vi "Building Array.vi"(0 "Vy array":dbl[](array[numeric]), 1 "Vx array":dbl[](array[numeric]), 2 "Timepoints":dbl[](array[numeric]), 3 "Folder to Save":path, 4 "No. of Gr":i32, 5 "No. of Sets":i32, 6 "Name of File":string, 7 "Folder Name":string) -> ()   [LabVIEW 2014]
uses:
  <vilib>/Utility/file.llb/Write Delimited Spreadsheet (DBL).vi
  <vilib>/Utility/file.llb/Read Delimited Spreadsheet (DBL).vi
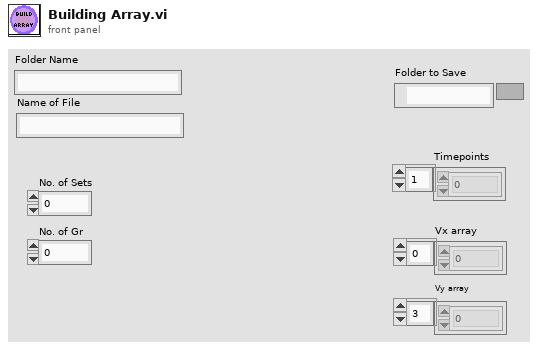
[diagram p1: front panel]
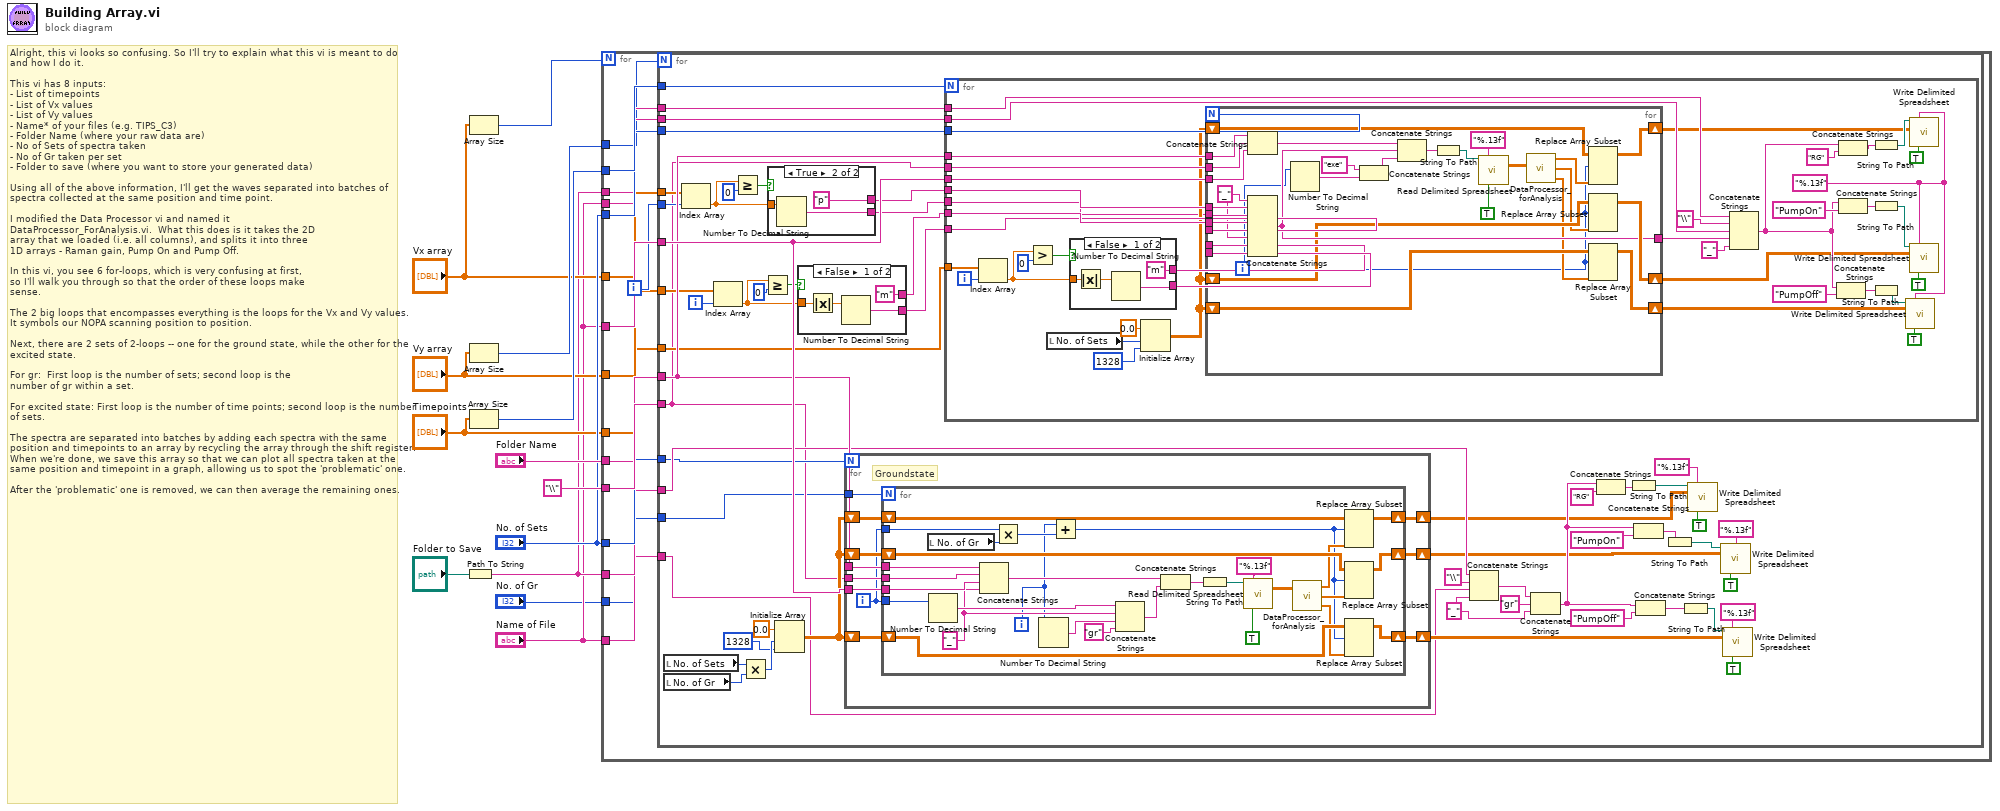
[diagram p0: block diagram]
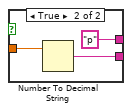
[diagram p2: hidden frame]
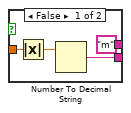
[diagram p3: hidden frame]
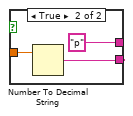
[diagram p4: hidden frame]
diagram:
  # "Alright, this vi looks so confusing. So I'll try to explain what this vi is meant to do and how I do it.\n\nThis vi has 8 inputs:\n- List of timepoints \n- List of Vx values \n- List of Vy values\n- Name* of your files (e.g. TIPS_C3)\n- Folder Name (where your raw data are)\n- No of Sets of spectra taken\n- No of Gr taken per set\n- Folder to save (where you want to store your generated data)\n\nUsing all of the above information, I'll get the waves separated into batches of spectra collected at the same position and time point.\n\nI modified the Data Processor vi and named it\nDataProcessor_ForAnalysis.vi.  What this does is it takes the 2D\narray that we loaded (i.e. all columns), and splits it into three\n1D arrays - Raman gain, Pump On and Pump Off.\n\nIn this vi, you see 6 for-loops, which is very confusing at first,\nso I'll walk you through so that the order of these loops make \nsense. \n\nThe 2 big loops that encompasses everything is the loops for the Vx and Vy values.  It symbols our NOPA scanning position to position.\n\nNext, there are 2 sets of 2-loops -- one for the ground state, while the other for the excited state.\n\nFor gr:  First loop is the number of sets; second loop is the\nnumber of gr within a set.\n\nFor excited state: First loop is the number of time points; second loop is the number of sets.\n\nThe spectra are separated into batches by adding each spectra with the same position and timepoints to an array by recycling the array through the shift register. When we're done, we save this array so that we can plot all spectra taken at the same position and timepoint in a graph, allowing us to spot the 'problematic' one. \n\nAfter the 'problematic' one is removed, we can then average the remaining ones."
  n1 = Path To String(path="Folder to Save") -> (string=w4:string)
  n2 = Array Size(array="Vx array") -> (size(s)=w2:i32)
  n3 = Array Size(array="Vy array") -> (size(s)=w11:i32)
  n4 = Array Size(array="Timepoints") -> (size(s)=w10:i32)
  n5 = for {
    N: w2 -> [_]
    tunnel: "Name of File" -> [w29]
    tunnel: "\\" -> [w28]
    tunnel: "Folder Name" -> [w27]
    tunnel: w11 -> [w15]
    tunnel: w10 -> [w26]
    tunnel: "No. of Sets" -> [w25]
    tunnel: "No. of Sets" -> [w24]
    tunnel: "Vx array" -> [w23]
    tunnel: "Vy array" -> [w21]
    tunnel: "Timepoints" -> [w20]
    tunnel: w4 -> [w19]
    tunnel: w4 -> [w18]
    tunnel: "Name of File" -> [w17]
    tunnel: "Name of File" -> [w16]
    tunnel: "No. of Gr" -> [w14]
    i -> [w22]
    n6 = for {
      N: w15 -> [_]
      tunnel: w29 -> [w84]
      tunnel: w28 -> [w36]
      tunnel: w27 -> [w83]
      tunnel: w26 -> [w82]
      tunnel: w25 -> [w81]
      tunnel: w24 -> [w39]
      tunnel: w23 -> [w77]
      tunnel: w22 -> [w78]
      tunnel: w21 -> [w73]
      tunnel: w20 -> [w67]
      tunnel: w19 -> [w66]
      tunnel: w18 -> [w65]
      tunnel: w17 -> [w32]
      tunnel: w16 -> [w49]
      tunnel: w14 -> [w35]
      i -> [w72]
      w45 = "_" ("string")
      n7 = local read "No. of Sets"() -> (w34:i32)
      n8 = local read "No. of Gr"() -> (w33:i32)
      n9 = Index Array(array=w77, index=w78) -> (element=w37:dbl)
      n10 = Index Array(array=w73, index=w72) -> (element=w74:dbl)
      n11 = Greater Or Equal?(x=w37, y=0) -> (x >= y?=w79:bool)
      n12 = Multiply(x=w34, y=w33) -> (x*y=w31:i32)
      n13 = Greater Or Equal?(x=w74, y=0) -> (x >= y?=w76:bool)
      n14 = case shown="True" w79 {
        tunnel: ["m" "p"] -> w71
        tunnel: w37 -> [w95 w96]
        tunnel: [w93 w97] -> w70
        frame False {
          n15 = Absolute Value(x=w95) -> (abs(x)=w94:dbl)
          n16 = Number To Decimal String(number=w94) -> (decimal integer string=w93:string)  [unwired: 1 in]
        }
        frame True {
          n17 = Number To Decimal String(number=w96) -> (decimal integer string=w97:string)  [unwired: 1 in]
        }
      }
      n18 = Initialize Array(0.0 ("element"), w31, 1328 ("dimension size")) -> (w38:dbl[][])
      n19 = case shown="False" w76 {
        tunnel: ["m" "p"] -> w69
        tunnel: w74 -> [w87 w89]
        tunnel: [w85 w90] -> w68
        frame False {
          n20 = Absolute Value(x=w87) -> (abs(x)=w86:dbl)
          n21 = Number To Decimal String(number=w86) -> (decimal integer string=w85:string)  [unwired: 1 in]
        }
        frame True {
          n22 = Number To Decimal String(number=w89) -> (decimal integer string=w90:string)  [unwired: 1 in]
        }
      }
      n23 = for {
        N: w39 -> [_]
        tunnel: w84 -> [w109]
        tunnel: w36 -> [w108]
        tunnel: w83 -> [w107]
        tunnel: w35 -> [w106]
        shift-right: [w105] -> w41
        shift-left: w38 -> [w102]
        shift-right: [w104] -> w43
        shift-left: w38 -> [w101]
        shift-right: [w103] -> w42
        shift-left: w38 -> [w100]
        i -> [w99]
        # "Groundstate"
        n24 = for {
          N: w106 -> [_]
          tunnel: w109 -> [w135]
          tunnel: w108 -> [w136]
          tunnel: w107 -> [w137]
          tunnel: w99 -> [w138]
          shift-right: [w119] -> w105
          shift-left: w102 -> [w118]
          shift-right: [w120] -> w103
          shift-left: w100 -> [w121]
          shift-right: [w123] -> w104
          shift-left: w101 -> [w122]
          tunnel: w99 -> [w116]
          i -> [w110]
          w133 = "_"
          n25 = local read "No. of Gr"() -> (w117:i32)
          n26 = Number To Decimal String(number=w138) -> (decimal integer string=w134:string)  [unwired: 1 in]
          n27 = Concatenate Strings(w137, w136, w135, w133) -> (w131:string)
          n28 = Multiply(x=w116, y=w117) -> (x*y=w115:i32)
          n29 = Number To Decimal String(number=w110) -> (decimal integer string=w132:string)  [unwired: 1 in]
          n30 = Add(x=w110, y=w115) -> (x+y=w111:i32)
          n31 = Concatenate Strings(w134, w133, w132, "gr" ("string")) -> (w124:string)
          n32 = Concatenate Strings(w131, w124) -> (w130:string)
          n33 = String To Path(string=w130) -> (path=w127:path)
          n34 = call-poly <vilib>:"Read Delimited Spreadsheet.vi"("file path (dialog if empty)"=w127, "format (%.3f)"="%.13f", "transpose? (F)"=TRUE) -> ("all rows"=w129:dbl[][])  [unwired: 7 in, 5 out]
          n35 = call "DataProcessor_forAnalysis.vi"("Data"=w129) -> ("PumpOff"=w113:dbl[], "PumpOn"=w114:dbl[], "Raman"=w112:dbl[])  [unwired: 3 in]
          n36 = Replace Array Subset(array=w118, new element=w112, index (row)=w111) -> (w119:dbl[][])  [unwired: 1 in]
          n37 = Replace Array Subset(array=w122, new element=w114, index (row)=w111) -> (w123:dbl[][])  [unwired: 1 in]
          n38 = Replace Array Subset(array=w121, new element=w113, index (row)=w111) -> (w120:dbl[][])  [unwired: 1 in]
        }
      }
      n39 = for {
        N: w82 -> [_]
        tunnel: w84 -> [w179]
        tunnel: w36 -> [w178]
        tunnel: w83 -> [w177]
        tunnel: w81 -> [w166]
        tunnel: w71 -> [w176]
        tunnel: w70 -> [w141]
        tunnel: w69 -> [w175]
        tunnel: w68 -> [w174]
        tunnel: w67 -> [w170]
        tunnel: w66 -> [w158]
        tunnel: w49 -> [w150]
        i -> [w169]
        w147 = "%.13f" ("format (%.3f)")
        n40 = Index Array(array=w170, index=w169) -> (element=w172:dbl)
        n41 = Greater?(x=w172, y=0) -> (0:w171:bool)
        n42 = local read "No. of Sets"() -> (w140:i32)
        n43 = case shown="False" w171 {
          tunnel: ["m" "p"] -> w167
          tunnel: w172 -> [w182 w184]
          tunnel: [w180 w185] -> w168
          frame False {
            n44 = Absolute Value(x=w182) -> (abs(x)=w181:dbl)
            n45 = Number To Decimal String(number=w181) -> (decimal integer string=w180:string)  [unwired: 1 in]
          }
          frame True {
            n46 = Number To Decimal String(number=w184) -> (decimal integer string=w185:string)  [unwired: 1 in]
          }
        }
        n47 = Initialize Array(0.0 ("element"), w140, 1328 ("dimension size")) -> (w142:dbl[][])
        n48 = for {
          N: w166 -> [_]
          tunnel: w179 -> [w207]
          tunnel: w178 -> [w198]
          tunnel: w177 -> [w197]
          tunnel: w176 -> [w213]
          tunnel: w141 -> [w212]
          tunnel: w175 -> [w211]
          tunnel: w174 -> [w210]
          tunnel: w168 -> [w209]
          tunnel: w167 -> [w200]
          shift-right: [w192] -> w144
          shift-left: w142 -> [w191]
          shift-right: [w194] -> w146
          shift-left: w142 -> [w195]
          shift-right: [w208] -> w145
          shift-left: w142 -> [w193]
          tunnel: [w201] -> w152
          i -> [w187]
          w199 = "_"
          n49 = Concatenate Strings(w197, w198, w207) -> (w206:string)
          n50 = Concatenate Strings(w199, w213, w212, w211, w210, w199, w200, w209) -> (w201:string)
          n51 = Number To Decimal String(number=w187) -> (decimal integer string=w204:string)  [unwired: 1 in]
          n52 = Concatenate Strings("exe", w204) -> (w203:string)
          n53 = Concatenate Strings(w206, w201, w203) -> (w202:string)
          n54 = String To Path(string=w202) -> (path=w214:path)
          n55 = call-poly <vilib>:"Read Delimited Spreadsheet.vi"("file path (dialog if empty)"=w214, "format (%.3f)"="%.13f", "transpose? (F)"=TRUE) -> ("all rows"=w216:dbl[][])  [unwired: 7 in, 5 out]
          n56 = call "DataProcessor_forAnalysis.vi"("Data"=w216) -> ("PumpOff"=w188:dbl[], "PumpOn"=w190:dbl[], "Raman"=w189:dbl[])  [unwired: 3 in]
          n57 = Replace Array Subset(array=w195, new element=w189, index (row)=w187) -> (w194:dbl[][])  [unwired: 1 in]
          n58 = Replace Array Subset(array=w193, new element=w190, index (row)=w187) -> (w208:dbl[][])  [unwired: 1 in]
          n59 = Replace Array Subset(array=w191, new element=w188, index (row)=w187) -> (w192:dbl[][])  [unwired: 1 in]
        }
        n60 = Concatenate Strings(w158, "\\" ("string"), w150, w152, "_" ("string")) -> (w148:string)
        n61 = Concatenate Strings(w148, "PumpOff") -> (w149:string)
        n62 = Concatenate Strings(w148, "RG") -> (w161:string)
        n63 = Concatenate Strings(w148, "PumpOn") -> (w159:string)
        n64 = String To Path(string=w161) -> (path=w160:path)
        n65 = String To Path(string=w159) -> (path=w156:path)
        n66 = String To Path(string=w149) -> (path=w155:path)
        n67 = call-poly <vilib>:"Write Delimited Spreadsheet.vi"("file path (dialog if empty)"=w155, "format (%.3f)"=w147, "2D data"=w144, "transpose? (F)"=TRUE) -> ()  [unwired: 10 in, 2 out]
        n68 = call-poly <vilib>:"Write Delimited Spreadsheet.vi"("file path (dialog if empty)"=w160, "format (%.3f)"=w147, "2D data"=w146, "transpose? (F)"=TRUE) -> ()  [unwired: 10 in, 2 out]
        n69 = call-poly <vilib>:"Write Delimited Spreadsheet.vi"("file path (dialog if empty)"=w156, "format (%.3f)"=w147, "2D data"=w145, "transpose? (F)"=TRUE) -> ()  [unwired: 10 in, 2 out]
      }
      n70 = Concatenate Strings(w65, "\\" ("string"), w32, w45) -> (w63:string)
      n71 = Concatenate Strings(w63, "gr" ("string"), w45) -> (w62:string)
      n72 = Concatenate Strings(w62, "RG") -> (w58:string)
      n73 = String To Path(string=w58) -> (path=w54:path)
      n74 = Concatenate Strings(w62, "PumpOn") -> (w57:string)
      n75 = Concatenate Strings(w62, "PumpOff") -> (w56:string)
      n76 = String To Path(string=w57) -> (path=w52:path)
      n77 = String To Path(string=w56) -> (path=w50:path)
      n78 = call-poly <vilib>:"Write Delimited Spreadsheet.vi"("file path (dialog if empty)"=w54, "format (%.3f)"="%.13f", "2D data"=w41, "transpose? (F)"=TRUE) -> ()  [unwired: 10 in, 2 out]
      n79 = call-poly <vilib>:"Write Delimited Spreadsheet.vi"("file path (dialog if empty)"=w52, "format (%.3f)"="%.13f", "2D data"=w43, "transpose? (F)"=TRUE) -> ()  [unwired: 10 in, 2 out]
      n80 = call-poly <vilib>:"Write Delimited Spreadsheet.vi"("file path (dialog if empty)"=w50, "format (%.3f)"="%.13f", "2D data"=w42, "transpose? (F)"=TRUE) -> ()  [unwired: 10 in, 2 out]
    }
  }
